vi "closeConnection_PubSub.vi"(8 "error in (no error)":errorcluster, 11 "LabVIEW-Python-Interface in":refnum<class "PyLVi.lvclass">) -> (0 "error out":errorcluster, 3 "LabVIEW-Python-Interface out":refnum<class "PyLVi.lvclass">)   [LabVIEW 2016, in "PyLVi.lvlib" / "PyLVi.lvclass"]
uses:
  PyLVi.lvclass
  PyLVi.lvclass/PyLVi.ctl
  <vilib>/addons/zeromq/zmq_socket.lvclass
  <vilib>/addons/zeromq/zmq_context.lvclass
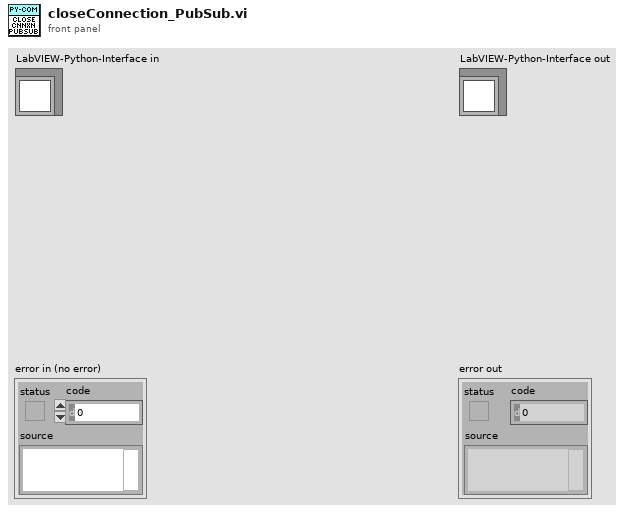
[diagram p1: front panel]
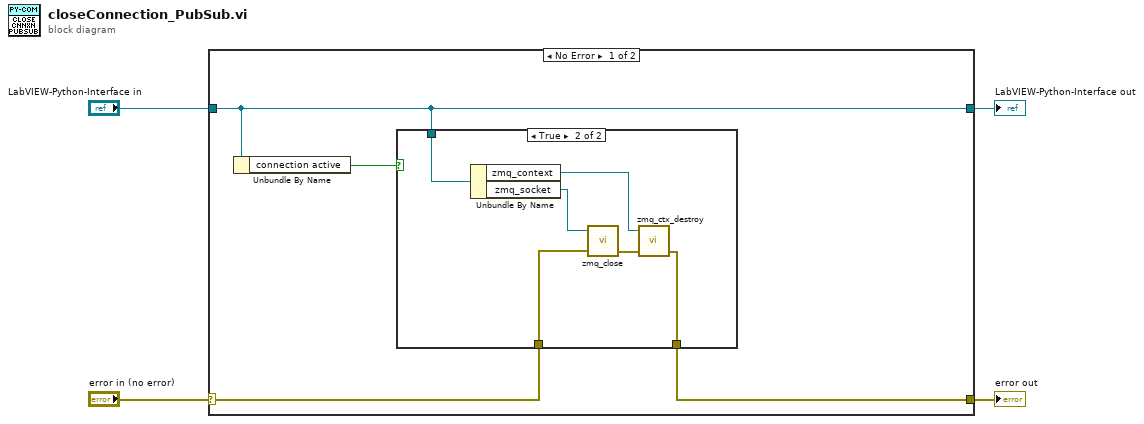
[diagram p0: block diagram]
diagram:
  n1 = case shown="No Error" "error in (no error)" {
    selector: "error in (no error)" -> [w7 w17]
    tunnel: [w8 w17] -> w3
    tunnel: [w6 w16] -> w1
    tunnel: "LabVIEW-Python-Interface in" -> [w6 w16]
    frame No Error {
      n2 = Unbundle By Name(w6) -> ("connection active"=w5:bool)
      n3 = case shown="True" w5 {
        tunnel: [w9 w14] -> w8
        tunnel: w7 -> [w9 w10]
        tunnel: w6 -> [_ w11]
        frame False {
        }
        frame True {
          n4 = Unbundle By Name(w11) -> ("zmq_context"=w12:refnum<class "zmq_context.lvclass">, "zmq_socket"=w13:refnum<class "zmq_socket.lvclass">)
          n5 = call <vilib>:"zmq_close.vi"("error in"=w10, "socket"=w13) -> ("error out"=w15:errorcluster)  [unwired: 3 in]
          n6 = call <vilib>:"zmq_ctx_destroy.vi"("error in"=w15, "context in"=w12) -> ("error out"=w14:errorcluster)  [unwired: 3 in]
        }
      }
    }
    frame Error {
    }
  }
  "error out" <- w3
  "LabVIEW-Python-Interface out" <- w1
